vi "CSM - Broadcast Event.vi"(6 "Auto Register? (T)":bool=TRUE, 8 "Error In":errorcluster caption="error in (no error)", 9 "Wait (5000ms)":i32=5000, 11 "CSM Module":string) -> (0 "error out":errorcluster, 1 "Waited (ms)":u32, 3 "Broadcast Event":T1)   [LabVIEW 2017, in "Communicable State Machine.lvlib"]
doc: "Obtains the CSM status change event refnum.\n\n-- <b>Controls</b> --\n- <b>CSM Module</b>: CSM module name.\n- <b>Wait (5000 ms)</b>: Timeout duration for waiting module to be alive. The default is 5000 ms.\n\n-- <b>Indicators</b> --\n- <b>Status Change Event</b>: CSM status change event refnum.\n- <b>Waited (ms)</b>: Time elapsed while waiting."
uses:
  Communicable State Machine.lvlib
  _Support/Typedef/_CSM Status Change Event Data.ctl
  _Support/CSMQ/_CSMOFGVOPER.ctl
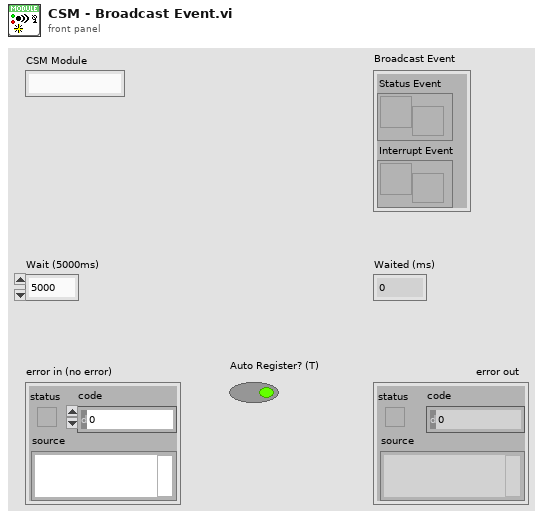
[diagram p1: front panel]
types:
  T1 = cluster{"Status Event":refnum<user-event>, "Interrupt Event":refnum<user-event>}
  T2 = typedef "Communicable State Machine.lvlib/_CSMOFGVOPER.ctl" = enum16{"Create If not Exist", "Get By Name", "List", "Check If Name Exists", "Release", "Module Status", "Create Status Event Handler", "Destroy Status Event Handler", "Clear Invalid Objs"}
  T3 = typedef "Communicable State Machine.lvlib/_CSMObj.ctl" = cluster{"info":T4, "Refs":T6}
  T4 = typedef "Communicable State Machine.lvlib/_CSMObj-Info.ctl" = cluster{"Module Name":string, "Requested Name":string, "Group Name":string, "Mode":T5, "Allowed Messages":string[]}
  T5 = typedef "Communicable State Machine.lvlib/_CSM_MODE.ctl" = enum16{"Not Exist", "Stand Alone", "CSM", "Worker", "Worker Agent", "Chain Node", "Chain"}
  T6 = typedef "Communicable State Machine.lvlib/_CSMObj-Refs.ctl" = cluster{"WatchDogQ":refnum<queue>, "CSMDataDVR":refnum<data-value>, "Queue":T7, "GroupDataDVR":refnum<data-value>, "TagMap":refnum<data-value>, "ExitEvent":refnum<user-event>, "NewStateEvent":refnum<user-event>, "StatusEvent":refnum<user-event>, "InterruptEvent":refnum<user-event>}
  T7 = typedef "Communicable State Machine.lvlib/Priority Queue.ctl" = cluster{"HPriorityQ":refnum<queue>, "LowPriorityQ":refnum<queue>}
  T8 = cluster{"StatusEvent":refnum<user-event>, "InterruptEvent":refnum<user-event>}
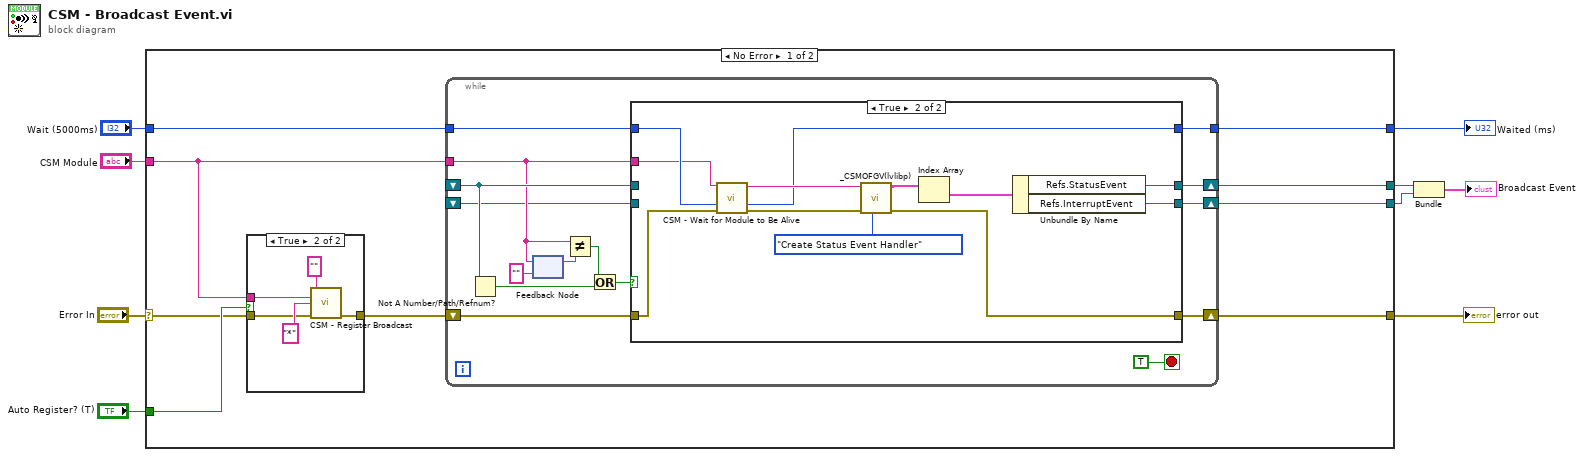
[diagram p0: block diagram]
diagram:
  n1 = case shown="No Error" "Error In" {
    selector: "Error In" -> [w12 w55]
    tunnel: [w18 _] -> w4
    tunnel: [w14 w55] -> w8
    tunnel: "CSM Module" -> [w10 _]
    tunnel: "Wait (5000ms)" -> [w17 _]
    tunnel: [w16 _] -> w5
    tunnel: [w15 _] -> w3
    tunnel: "Auto Register? (T)" -> [w13 _]
    frame No Error {
      n2 = case shown="True" w13 {
        tunnel: w12 -> [w19 w22]
        tunnel: [w19 w21] -> w11
        tunnel: w10 -> [_ w20]
        frame False {
        }
        frame True {
          n3 = call "CSM - Register Broadcast.vi"("CSM Name(Empty for Broadcast Event)"="" ("CSM Name"), "Source CSM Name (* as Default)"=w20, "Trigger"="*" ("CSM Name"), "Error In"=w22) -> ("error out"=w21:errorcluster)  [unwired: 10 in, 1 out]
        }
      }
      n4 = while {
        shift-right: [w37] -> w14
        shift-left: w11 -> [w38]
        shift-right: [w39] -> w18
        shift-left: _ -> [w35]
        tunnel: w10 -> [w33]
        tunnel: w17 -> [w28]
        tunnel: [w27] -> w16
        shift-right: [w26] -> w15
        shift-left: _ -> [w25]
        stop <- TRUE stop-if-true
        n5 = Not A Number/Path/Refnum?(number/path/refnum=w35) -> (NaN/Path/Refnum?=w31:bool)
        n6 = feedback-in #1(w33) -> ()
        n7 = feedback #1("" ("CSM Module")) -> (w32:string)
        n8 = Not Equal?(x=w33, y=w32) -> (x != y?=w30:bool)
        n9 = Or(x=w30, y=w31) -> (x .or. y?=w34:bool)
        n10 = case shown="True" w34 {
          tunnel: [w42 w50] -> w39
          tunnel: w38 -> [w41 w49]
          tunnel: [w41 w53] -> w37
          tunnel: w35 -> [w42 _]
          tunnel: w33 -> [_ w45]
          tunnel: w28 -> [_ w46]
          tunnel: [_ w44] -> w27
          tunnel: [w40 w43] -> w26
          tunnel: w25 -> [w40 _]
          frame False {
          }
          frame True {
            n11 = call "CSM - Wait for Module to Be Alive.vi"("CSM Name"=w45, "Wait (5000 ms)"=w46, "error in (no error)"=w49) -> ("CSM Name (Dup)"=w47:string, "Waited (ms)"=w44:u32, "error out"=w48:errorcluster)  [unwired: 10 in]
            n12 = call "_CSMOFGV(lvlibp).vi"("Operation"=_CSMOFGVOPER."Create Status Event Handler", "Error In"=w48, "Name (\"\" to Use UUID) In"=w47) -> ("error out"=w53:errorcluster, "Array"=w52:T3[])  [unwired: 6 in, 1 out]
            n13 = Index Array(array=w52) -> (element=w51:T3)  [unwired: 1 in]
            n14 = Unbundle By Name(w51) -> ("Refs.StatusEvent"=w50:refnum<user-event>, "Refs.InterruptEvent"=w43:refnum<user-event>)
          }
        }
      }
    }
    frame Error {
    }
  }
  "error out" <- w8
  "Waited (ms)" <- w5
  n15 = Bundle("StatusEvent"=w4, "InterruptEvent"=w3) -> (→"Broadcast Event":T8)  [unwired: 1 in]
